vi "Send Stop.vi"(7 "Emergency Stop? (F)":bool, 8 "error in (no error)":errorcluster, 11 "Actor Interface in":refnum<data-value>) -> (0 "error out":errorcluster, 3 "Actor Interface out":refnum<data-value>)   [LabVIEW 2018, in "Actor.lvlib" / "Actor-Interface.lvclass"]
uses:
  Actor-Interface.lvclass
  Actor-Interface.lvclass/Actor-Interface.ctl
  Stop.ctl
  <vilib>/event_ctls.llb/usereventprio.ctl
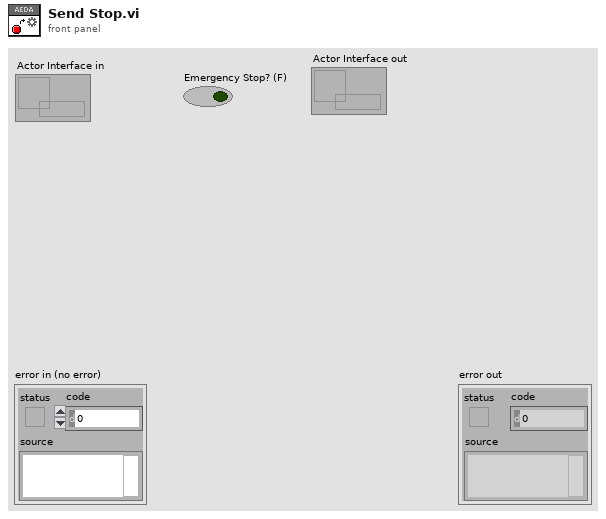
[diagram p1: front panel]
types:
  T1 = typedef "Actor.lvlib/Actor-Interface.lvclass/Stop.ctl" = enum16{"Normal", "Emergency"}
  T2 = typedef "usereventprio.ctl" = enum32{"high priority", "normal priority"}
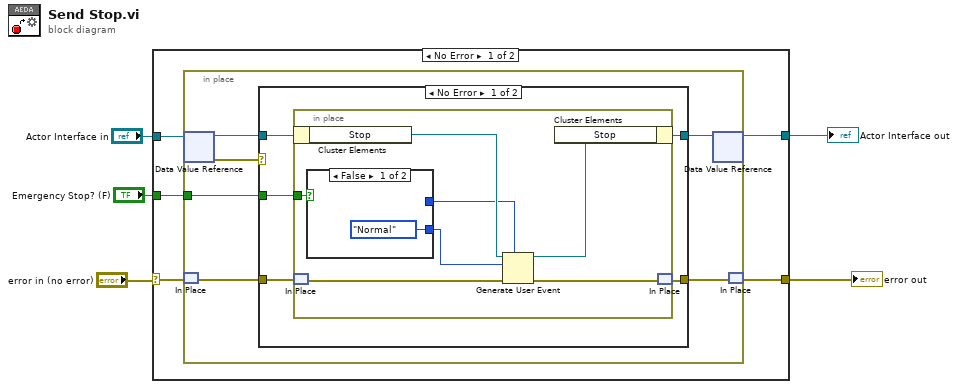
[diagram p0: block diagram]
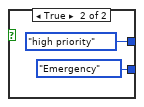
[diagram p2: hidden frame]
diagram:
  n1 = case shown="No Error" "error in (no error)" {
    selector: "error in (no error)" -> [w9 w35]
    tunnel: [w8 w35] -> w2
    tunnel: [w7 w34] -> w1
    tunnel: "Actor Interface in" -> [w10 w34]
    tunnel: "Emergency Stop? (F)" -> [w6 _]
    frame No Error {
      n2 = in-place {
        in-place-border: w6 -> [w11]
        n3 = in-place-dvr #1(w10) -> (w15:refnum<class "Actor-Interface.lvclass">, w16:errorcluster)
        n4 = in-place-match #2(w9) -> (w13:errorcluster)
        n5 = case shown="No Error" w16 {
          selector: w16 -> [_ w33]
          tunnel: w15 -> [w19 w32]
          tunnel: [w17 w32] -> w14
          tunnel: w13 -> [w21 _]
          tunnel: [w20 w33] -> w12
          tunnel: w11 -> [w18 _]
          frame No Error {
            n6 = in-place {
              in-place-border: w18 -> [w26]
              n7 = in-place-cluster #3(w19) -> ("Stop"=w27:refnum<user-event>)
              n8 = in-place-match #4(w21) -> (w28:errorcluster)
              n9 = case shown="False" w26 {
                tunnel: [Stop."Normal" ("Stop") Stop."Emergency" ("Stop")] -> w24
                tunnel: [_ usereventprio."high priority" ("priority (normal)")] -> w23
                frame False {
                }
                frame True {
                }
              }
              n10 = Generate User Event(priority (normal)=w23, user event=w27, event data cluster=w24, error in=w28) -> (user event out=w25:refnum<user-event>, error out=w22:errorcluster)
              n11 = in-place-cluster #3("Stop"=w25) -> (w17:refnum<class "Actor-Interface.lvclass">)
              n12 = in-place-match #4(w22) -> (w20:errorcluster)
            }
          }
          frame Error {
          }
        }
        n13 = in-place-dvr #1(w14) -> (w7:refnum<data-value>)  [unwired: 1 out]
        n14 = in-place-match #2(w12) -> (w8:errorcluster)
      }
    }
    frame Error {
    }
  }
  "error out" <- w2
  "Actor Interface out" <- w1
